vi "Sequence.Test.DMC.GetComponent.vi"(6 "TS (now)":timestamp, 7 "Default":bool, 8 "Cnt (0)":i32, 9 "Component":T7, 10 "Plate":T1, 11 "OrderSets":T2={"State"=enum."Init", "ImgPath"=path "", "WabcoPlate"="", "WabcoProduct"="", "ClientProduct"="", "ClientPlate"="", "TotalQuantity"=0, "OrderQuantity"=0, "Serial"=0, "Wabco"={"LaserJob"="", "AdditionalTxt"="037", "FactoryCode"="", "RevID"=0, "ForkID"=0, "FailuresLimit"=0, "GlobalCnt"=0, "Bank"=0, "SerialFormat"=enum."6 dig", "CoordA"={"X"=0.0, "Y"=0.0, "Angle"=0.0}, "CoordB"={"X"=0.0, "Y"=0.0, "Angle"=0.0}, "DMCconfig"=0}, "Client"={"LaserJob"="", "AdditionalTxt"="", "FactoryCode"="037", "RevID"=0, "ForkID"=0, "FailuresLimit"=0, "GlobalCnt"=0, "Bank"=0, "SerialFormat"=enum."6 dig", "CoordA"={"X"=0.0, "Y"=0.0, "Angle"=0.0}, "CoordB"={"X"=0.0, "Y"=0.0, "Angle"=0.0}, "DMCconfig"=0}}) -> (1 "max size":i32, 2 "size":i32, 3 "Value":string)   [LabVIEW 2016]
uses:
  Gui/DMCConfiguatorGui.Component.ctl
  Gui/DMCConfiguatorGui.Type.ctl
  Gui/DMCConfiguatorGui.Var.ctl
  Logger/Logger.Variant.Sets.ctl
  Station/Station.Changeover.State.vi
  Station/Station.Plate.Properties.ctl
  Sequence.Code.SerialFormat.ctl
  Drivers/V7310/LowLevel/V7310.Job.Sets.ctl
  Sequence.PlateType.ctl
  Drivers/V7310/LowLevel/V7310.Global.vi
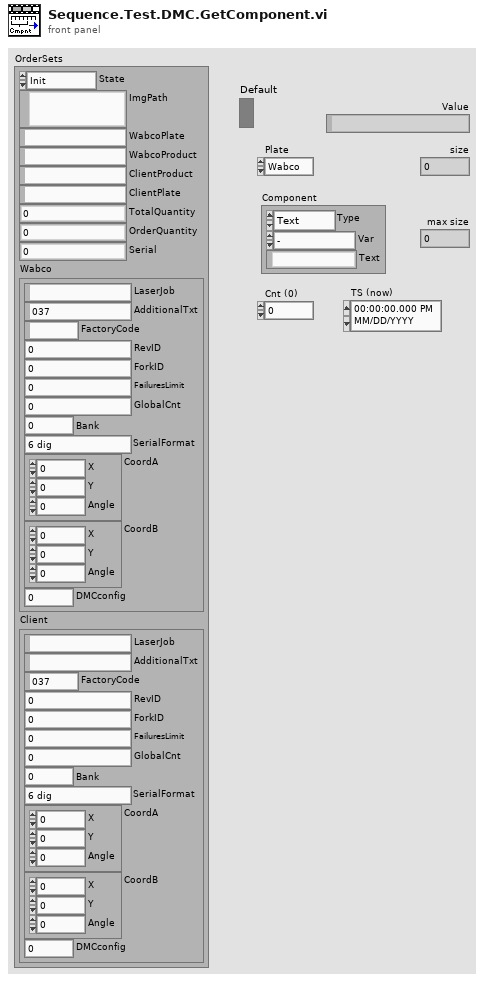
[diagram p1: front panel]
types:
  T1 = typedef "Sequence.PlateType.ctl" = enum16{"Wabco", "Client"}
  T2 = typedef "Logger.Variant.Sets.ctl" = cluster{"State":T3, "ImgPath":path, "WabcoPlate":string, "WabcoProduct":string, "ClientProduct":string, "ClientPlate":string, "TotalQuantity":u16, "OrderQuantity":u16, "Serial":i32, "Wabco":T4, "Client":T4}
  T3 = typedef "Station.Changeover.State.vi" = enum16{"Init", "Scaning", "NOK", "Wait for ack", "Ready"}
  T4 = typedef "Station.Plate.Properties.ctl" = cluster{"LaserJob":string, "AdditionalTxt":string, "FactoryCode":string, "RevID":u8, "ForkID":u8, "FailuresLimit":u16, "GlobalCnt":i32, "Bank":u8, "SerialFormat":T5, "CoordA":T6, "CoordB":T6, "DMCconfig":i32}
  T5 = typedef "Sequence.Code.SerialFormat.ctl" = enum8{"", "6 dig", "7 dig"}
  T6 = typedef "V7310.Job.Sets.ctl" = cluster{"X":dbl, "Y":dbl, "Angle":dbl}
  T7 = typedef "DMCConfiguatorGui.Component.ctl" = cluster{"Type":T8, "Var":T9, "Text":string}
  T8 = typedef "DMCConfiguatorGui.Type.ctl" = enum8{"Text", "Variable"}
  T9 = typedef "DMCConfiguatorGui.Var.ctl" = enum8{"-", "Wabco No", "Client No", "Serial", "Date"}
  T10 = typedef "V7310.Data.Status.ctl" = cluster{"State":T11, "LaserStatus":T12, "LaserStatusRaw":string, "Ref":refnum<k5>, "RTC TS":timestamp, "Conn TS":timestamp, "Msg":T13[], "JobInUse":string, "Jobs":string[], "Vars":T14[]}
  T11 = typedef "V7310.Data.Status.State.ctl" = enum16{"First", "Init", "Msg", "Error", "Abort", "Idle", "Run"}
  T12 = typedef "V7310.LaserStatus.ctl" = enum16{"-", "FatalError", "Initialize", "KeySwitchOpen", "TimeoutInterlock", "InterlockOpen", "StartUp", "ShutterlockOpen", "Standby", "Ready", "PrepareForMarking", "WaitForTrigger", "Marking"}
  T13 = typedef "V7310.Message.Data.ctl" = cluster{"ID":i32, "Msg":string}
  T14 = typedef "V7310.Job.Variable.ctl" = cluster{"Name":string, "Value":string}
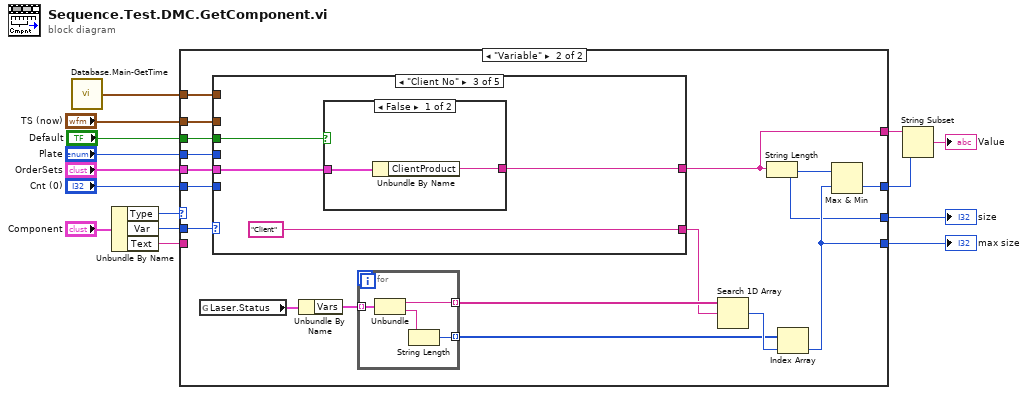
[diagram p0: block diagram]
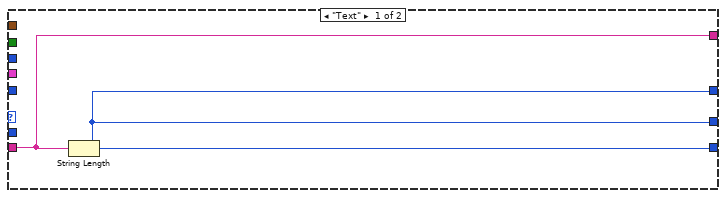
[diagram p2: hidden frame]
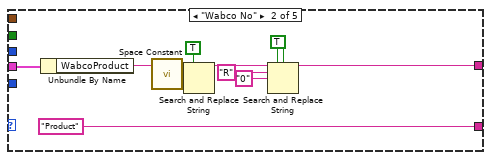
[diagram p4: hidden frame]
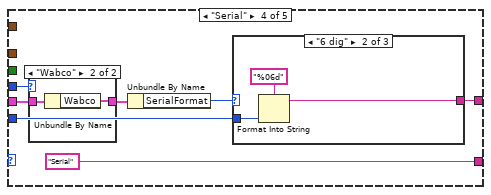
[diagram p6: hidden frame]
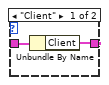
[diagram p7: hidden frame]
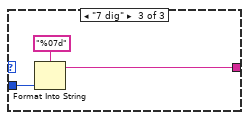
[diagram p9: hidden frame]
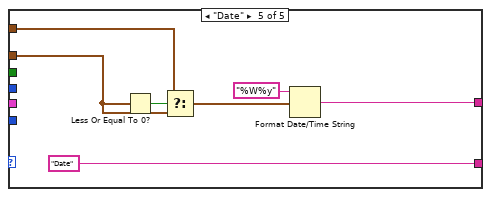
[diagram p10: hidden frame]
diagram:
  n1 = call "Database.Main-GetTime.vi"() -> ("TS"=w1:timestamp)  [unwired: 1 in]
  n2 = Unbundle By Name("Component") -> ("Type"=w14:T8, "Var"=w12:T9, "Text"=w13:string)
  n3 = case shown="\"Variable\"" w14 {
    tunnel: w13 -> [w17 _]
    tunnel: w12 -> [_ w29]
    tunnel: [w16 w25] -> w11
    tunnel: "OrderSets" -> [_ w27]
    tunnel: [w16 w23] -> w7
    tunnel: "Plate" -> [_ w26]
    tunnel: [w17 w24] -> w8
    tunnel: "Cnt (0)" -> [_ w22]
    tunnel: "TS (now)" -> [_ w21]
    tunnel: "Default" -> [_ w20]
    tunnel: [w16 w19] -> w2
    tunnel: w1 -> [_ w18]
    frame "Text" {
      n4 = String Length(string=w17) -> (length=w16:i32)
    }
    frame "Variable" {
      n5 = global read "V7310.Global.vi" "Laser.Status"() -> (w34:T10)
      n6 = case shown="\"Client No\"" w29 {
        tunnel: [_ "Product" ("element") "Client" ("element") "Serial" ("element") "Date" ("element")] -> w28
        tunnel: w27 -> [_ w40 w47 w56 _]
        tunnel: [_ w35 w46 w52 w73] -> w24
        tunnel: w26 -> [_ _ _ w53 _]
        tunnel: w22 -> [_ _ _ w51 _]
        tunnel: w21 -> [_ _ _ _ w70]
        tunnel: w20 -> [_ _ w45 _ _]
        tunnel: w18 -> [_ _ _ _ w68]
        frame "-" {
        }
        frame "Wabco No" {
          w37 = TRUE ("replace all? (F)")
          n7 = Unbundle By Name(w40) -> ("WabcoProduct"=w41:string)
          n8 = call <vilib>:"Space Constant.vi"() -> ("String"=w43:string)
          n9 = Search and Replace String(replace all?=TRUE ("replace all? (F)"), input string=w41, search string=w43) -> (result string=w36:string)  [unwired: 5 in, 3 out]
          n10 = Search and Replace String(replace all?=w37, case sensitive?=w37, input string=w36, search string="R", replace string="0" ("replace string (\"\")")) -> (result string=w35:string)  [unwired: 3 in, 3 out]
        }
        frame "Client No" {
          n11 = case shown="False" w45 {
            tunnel: w47 -> [w50 _]
            tunnel: [w49 _] -> w46
            frame False {
              n12 = Unbundle By Name(w50) -> ("ClientProduct"=w49:string)
            }
            frame True {
            }
          }
        }
        frame "Serial" {
          n13 = case shown="\"Wabco\"" w53 {
            tunnel: w56 -> [w59 w61]
            tunnel: [w58 w60] -> w55
            frame "Client" {
              n14 = Unbundle By Name(w59) -> ("Client"=w58:T4)
            }
            frame "Wabco" {
              n15 = Unbundle By Name(w61) -> ("Wabco"=w60:T4)
            }
          }
          n16 = Unbundle By Name(w55) -> ("SerialFormat"=w54:T5)
          n17 = case shown="\"6 dig\"" w54 {
            tunnel: w51 -> [_ w64 w67]
            tunnel: [_ w62 w65] -> w52
            frame "" {
            }
            frame "6 dig" {
              n18 = Format Into String(format string="%06d", w64) -> (resulting string=w62:string)  [unwired: 2 in, 1 out]
            }
            frame "7 dig" {
              n19 = Format Into String(format string="%07d", w67) -> (resulting string=w65:string)  [unwired: 2 in, 1 out]
            }
          }
        }
        frame "Date" {
          n20 = Less Or Equal To 0?(x=w70) -> (x <= 0?=w71:bool)
          n21 = Select(t=w68, s=w71, f=w70) -> (s? t:f=w69:timestamp)
          n22 = Format Date/Time String(time format string (%c)="%W%y", seconds (now)=w69) -> (date/time string=w73:string)  [unwired: 1 in]
        }
      }
      n23 = Unbundle By Name(w34) -> ("Vars"=w33:T14[])
      n24 = for {
        tunnel: w33 -> [w78] mode=indexing
        tunnel: [w77] -> w31 mode=indexing
        tunnel: [w75] -> w30 mode=indexing
        n25 = Unbundle(w78) -> ("Name"=w77:string, "Value"=w76:string)
        n26 = String Length(string=w76) -> (length=w75:i32)
      }
      n27 = Search 1D Array(1D array=w31, element=w28) -> (index of element=w32:i32)  [unwired: 1 in]
      n28 = String Length(string=w24) -> (length=w19:i32)
      n29 = Index Array(array=w30, index=w32) -> (element=w25:i32)
      n30 = Max & Min(x=w19, y=w25) -> (min(x,y)=w23:i32)  [unwired: 1 out]
    }
  }
  "max size" <- w11
  "size" <- w2
  n31 = String Subset(string=w8, length (rest)=w7) -> (substring=→"Value":string)  [unwired: 1 in]
